vi "Stack.vi"(10 "stack?":bool) -> ()   [LabVIEW 2014]
uses:
  <vilib>/Rock Robotics/WPI/Solenoid/WPI_SolenoidValue.ctl
  <vilib>/Rock Robotics/WPI/Solenoid/WPI_SolenoidSetEnum.vi
  Robot Global Data.vi
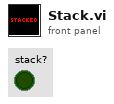
[diagram p1: front panel]
types:
  T1 = typedef "WPI_SolenoidValue.ctl" = enum16{"Off", "On", "Forward", "Reverse"}
  T2 = typedef "WPI_SolenoidDevRef.ctl" = cluster{"DevStatus":errorcluster, "Pneumatics Control Module":u8, "Forward Solenoid Channel":T3, "Reverse Solenoid Channel":T3}
  T3 = typedef "WPI_SolenoidChannel.ctl" = enum8{"Solenoid 0", "Solenoid 1", "Solenoid 2", "Solenoid 3", "Solenoid 4", "Solenoid 5", "Solenoid 6", "Solenoid 7", "Invalid"}
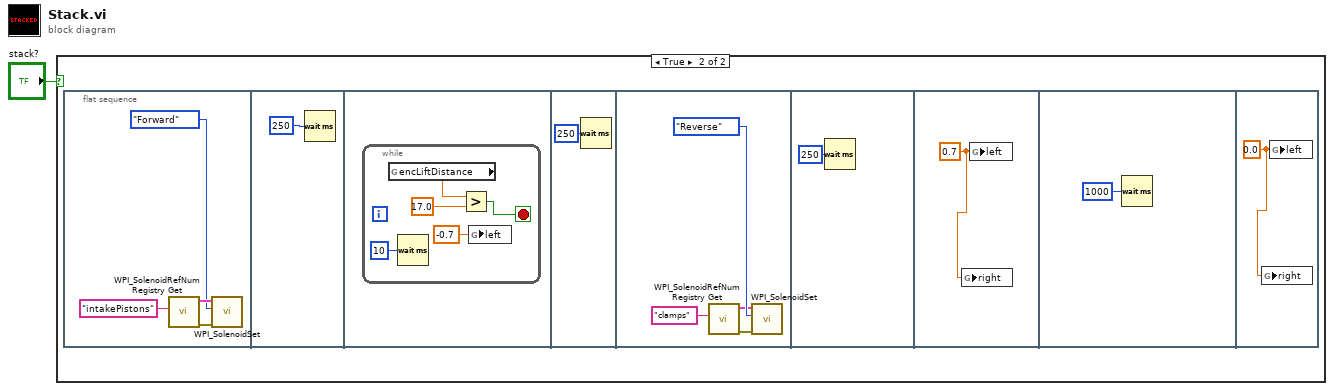
[diagram p0: block diagram]
diagram:
  n1 = case shown="True" "stack?" {
    frame False {
    }
    frame True {
      n2 = flat-sequence {
        frame #0 {
          n3 = call <vilib>:"WPI_SolenoidRefNum Registry Get.vi"("refnum name"="intakePistons") -> ("error out"=w3:errorcluster, "SolenoidDevRef"=w4:T2)  [unwired: 9 in]
          n4 = call-poly <vilib>:"WPI_SolenoidSet.vi"("error in (no error)"=w3, "Value"=WPI_SolenoidValue."Forward", "SolenoidDevRef"=w4) -> ()  [unwired: 7 in, 2 out]
        }
        frame #1 {
          n5 = Wait (ms)(milliseconds to wait=u32 250) -> ()  [unwired: 1 out]
        }
        frame #2 {
          n6 = while {
            stop <- w10 stop-if-true
            n7 = global read "Robot Global Data.vi" "encLiftDistance"() -> (w9:dbl)
            n8 = Wait (ms)(milliseconds to wait=u32 10) -> ()  [unwired: 1 out]
            n9 = Greater?(x=w9, y=17.0) -> (0:w10:bool)
            n10 = global write "Robot Global Data.vi" "left"(-0.7 ("left")) -> ()
          }
        }
        frame #3 {
          n11 = Wait (ms)(milliseconds to wait=u32 250) -> ()  [unwired: 1 out]
        }
        frame #4 {
          n12 = call <vilib>:"WPI_SolenoidRefNum Registry Get.vi"("refnum name"="clamps") -> ("error out"=w15:errorcluster, "SolenoidDevRef"=w14:T2)  [unwired: 9 in]
          n13 = call-poly <vilib>:"WPI_SolenoidSet.vi"("error in (no error)"=w15, "Value"=WPI_SolenoidValue."Reverse", "SolenoidDevRef"=w14) -> ()  [unwired: 7 in, 2 out]
        }
        frame #5 {
          n14 = Wait (ms)(milliseconds to wait=u32 250) -> ()  [unwired: 1 out]
        }
        frame #6 {
          w18 = 0.7 ("left")
          n15 = global write "Robot Global Data.vi" "right"(w18) -> ()
          n16 = global write "Robot Global Data.vi" "left"(w18) -> ()
        }
        frame #7 {
          n17 = Wait (ms)(milliseconds to wait=u32 1000) -> ()  [unwired: 1 out]
        }
        frame #8 {
          w20 = 0.0 ("left")
          n18 = global write "Robot Global Data.vi" "right"(w20) -> ()
          n19 = global write "Robot Global Data.vi" "left"(w20) -> ()
        }
      }
    }
  }
